vi "Calibration_user_input.vi"(4 "data mode":enum16{"Take new data point", "Refit Curve"}(ring), 6 "Mode":T4, 7 "Fixed n":bool, 8 "OK":T13, 9 "Sampling speeds":T5={"Samples /ch"=300, "Sampling Rate /ch (Hz)"=50.0} {"Sampling Rate /ch (Hz)" min=0 format="%.2f"; "Samples /ch" min=0 step=1}) -> (1 "Sampling speeds Output":T5={"Samples /ch"=300, "Sampling Rate /ch (Hz)"=50.0} {"Sampling Rate /ch (Hz)" min=0 format="%.2f"; "Samples /ch" min=0 step=1}, 2 "Fixed n out":bool, 3 "Temp":dbl=21.0 format="%.1fC", 5 "Abs Press":dbl=1013.0 format="%.1fmBar")   [LabVIEW 2022 SP3]
uses:
  Controls/ok_button.ctl
  Calib Channel Setup.ctl
  Controls/Cal_Inst_type.ctl
  Controls/Ref_Inst_type.ctl
  Calib_mode.ctl
  Controls/PWA_Data.ctl
  Controls/zeroableInst.ctl
  Controls/Meas input Cluster.ctl
  Controls/Inst_type.ctl
  Controls/portOrDev.ctl
  Controls/calType.ctl
  Controls/channelState.ctl
  File/Setup_Filetype.ctl
  ADAM Client/Sub VIs/ADAM Controls/Channel_names.ctl
  <vilib>/Utility/error.llb/Trim Whitespace One-Sided.vi
  Globals/Calib_global.vi
  Globals/Constants_global.vi
  Globals/Meas_global.vi
panel:
  in  "zeroable?":T1
  out "InstADAMChName":string
  in  "Select ADAM Instrument":bool
  in  "PWA Data":T2
  in  "Ref Instrument type":T3
  out "Info":string
  out "XW Angle Calib Present?":bool
  out "XW Velocity Calib Present?":bool
  in  "Edit temp and Press":bool
  out "2nd ref instrument":T6={"2nd Ref type"=enum."LDA", "2nd inst present"=TRUE}
  in  "Ref vel for angle calib":T7={"Ch"=4, "Off ch no"=0, "Calib filename"=path "", "Ref Instrument type"=enum."LDA", "DAQ System"="", "Port/Dev"=""} {"Off ch no" min=0 max=1; "Ch" min=0 max=50}
  out "Instrument type":T8=enum."Cross wire angle"
  in  "angle calib":T9(ring)
  in  "Reference instrument":T10={"Ch"=4, "Off ch no"=0, "Calib filename"=path "", "Ref Instrument type"=enum."Enter Value", "Device"="", "Port"=""} {"Off ch no" min=0 max=1; "Ch" min=0 max=50}
  in  "instrument to calibrate":T11(array[cluster])=[{"Ch No"=1, "Off ch no"=1, "Acquisition Plug in "="", "Port"=""}, {"Ch No"=2, "Off ch no"=1, "Acquisition Plug in "="", "Port"=""}] {"Off ch no" min=0 max=1; "Ch No" min=0 max=1000}
  in  "Instrument type":T8=enum."Pressure Transducer"
  out "Calib filename":path
  out "Ch & spans":T12[](array[typedef])=[{"Ch No"=1, "Var name"="Cross wire 1", "Device"="", "Port"=""}, {"Ch No"=2, "Var name"="Cross wire 2", "Device"="", "Port"=""}] {"Ch No" min=0 max=7}
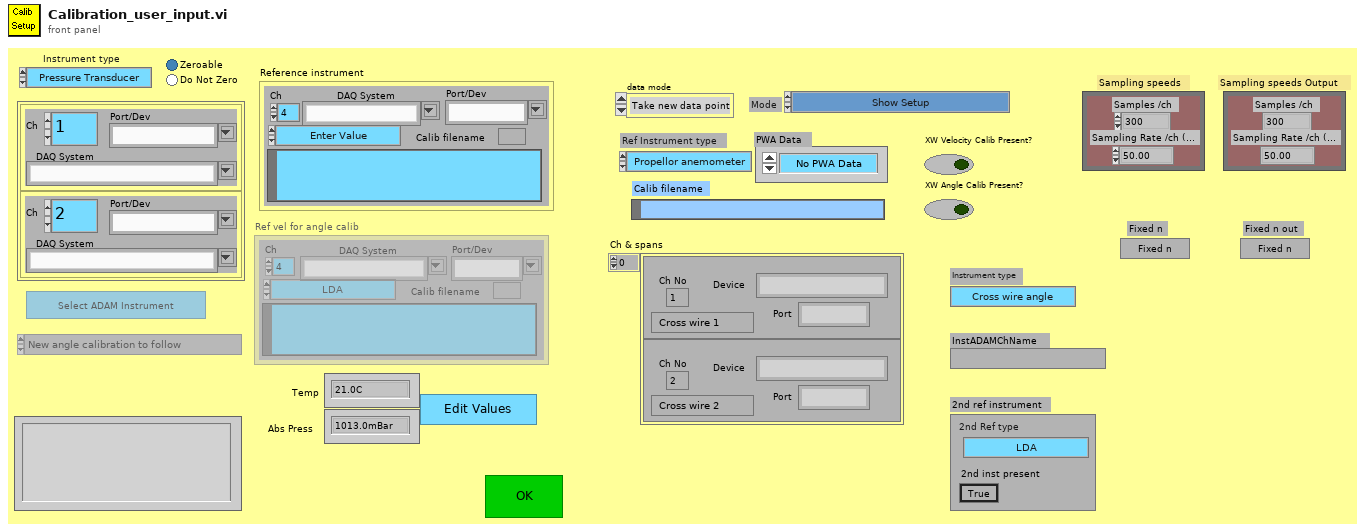
[diagram p1: front panel]
types:
  T1 = typedef "zeroableInst.ctl" = enum32{"Zeroable", "Do Not Zero"}
  T2 = typedef "PWA_Data.ctl" = enum16{"No PWA Data", "One Ch PWA"}
  T3 = typedef "Ref_Inst_type.ctl" = enum16{"Propellor anemometer", "Pressure Transducer", "Raw voltage", "Pitot-static tube", "Generic Linear", "Generic Polynomial", "Thermocouple", "LDA", "Enter Value", "ADAM Channel"}
  T4 = typedef "Calib_mode.ctl" = enum16{"Show Setup", "Take a New Calibration Point", "Refit Curve", "Setup Front Panel"}
  T5 = cluster{"Samples /ch":i32, "Sampling Rate /ch (Hz)":sgl}
  T6 = cluster{"2nd Ref type":T3, "2nd inst present":bool}
  T7 = cluster{"Ch":i16, "Off ch no":i8, "Calib filename":path, "Ref Instrument type":T3, "DAQ System":string, "Port/Dev":string}
  T8 = typedef "Cal_Inst_type.ctl" = enum16{"Propeller anemometer", "Pressure Transducer", "Hot wire", "Cross wire velocity", "Cross wire angle", "Generic Linear", "Generic Polynomial", "Poly Fit Special", "Fast FID", "Thermocouple", "Cold wire", "Pulsed Wire"}
  T9 = enum16{"New angle calibration to follow", "Use the most recent angle calibration"}
  T10 = cluster{"Ch":i16, "Off ch no":i8, "Calib filename":path, "Ref Instrument type":T3, "Device":string, "Port":string}
  T11 = cluster{"Ch No":i16, "Off ch no":i8, "Acquisition Plug in ":string, "Port":string}[]
  T12 = typedef "Calib Channel Setup.ctl" = cluster{"Ch No":i16, "Var name":string, "Device":string, "Port":string}
  T13 = typedef "ok_button.ctl" = bool
  T14 = typedef "Meas input Cluster.ctl" = cluster{"Type":T15, "Label":string, "DAQ":string, "Port":T16, "Ch":i32, "Cal":path, "calType":T17, "Fs":dbl, "syncDelay":dbl, "chState":T18}
  T15 = typedef "Inst_type.ctl" = enum16{"Raw voltage", "Raw with zero offsetting", "Propeller anemometer", "Pressure Transducer", "Pitot-static tube", "Hot wire", "Cross wire 1", "Cross wire 2", "Generic Linear", "Generic Polynomial", "Generic BackPoly", "Fast FID", "Thermocouple", "Cold wire", "Pulsed Wire", "LDA Vel", "LDA Tran time", "LDA Arr time", "Microphone"}
  T16 = typedef "portOrDev.ctl" = string
  T17 = typedef "calType.ctl" = enum32{"Latest", "Fixed"}
  T18 = typedef "channelState.ctl" = enum32{"No Selection", "Solo", "Mute"}
  T19 = typedef "Setup_Filetype.ctl" = enum16{"Measurement Setups", "Calibration Setups", "General", "Results File Plotter Setups", "Speed Calib Tweaks"}
  T20 = enum8{"Enabled", "Disabled", "Disabled and Grayed Out"}
  T21 = typedef "Channel_names.ctl" = enum16{"Active Only", "Active + Off", "All Channels", "Changeable Only", "Always Off", "Always On", "Always Off or On"}
  T22 = cluster{"Ch No":i16, "Off ch no":i8, "Device":string, "Port":string}[]
  T23 = cluster{"Ch No":i16, "Off ch no":i8, "Acquisition Plug in ":string, "Port":string}
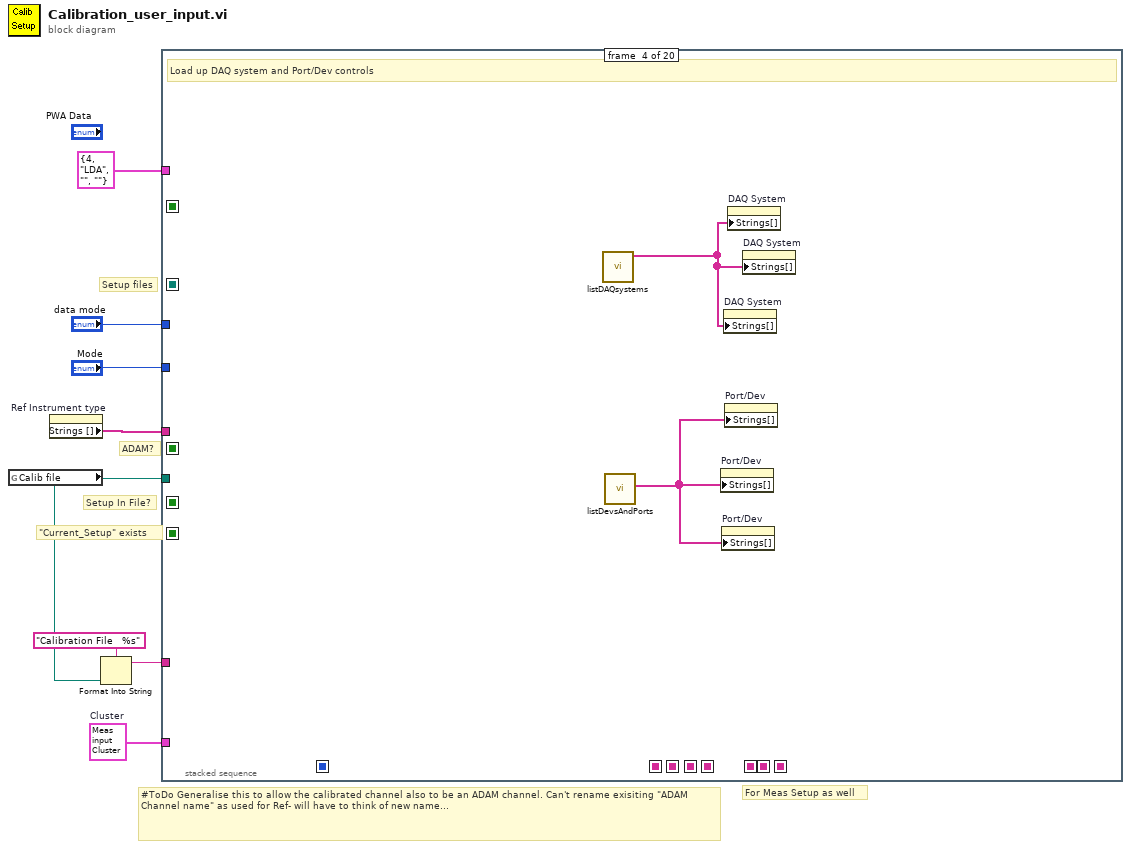
[diagram p0: block diagram]
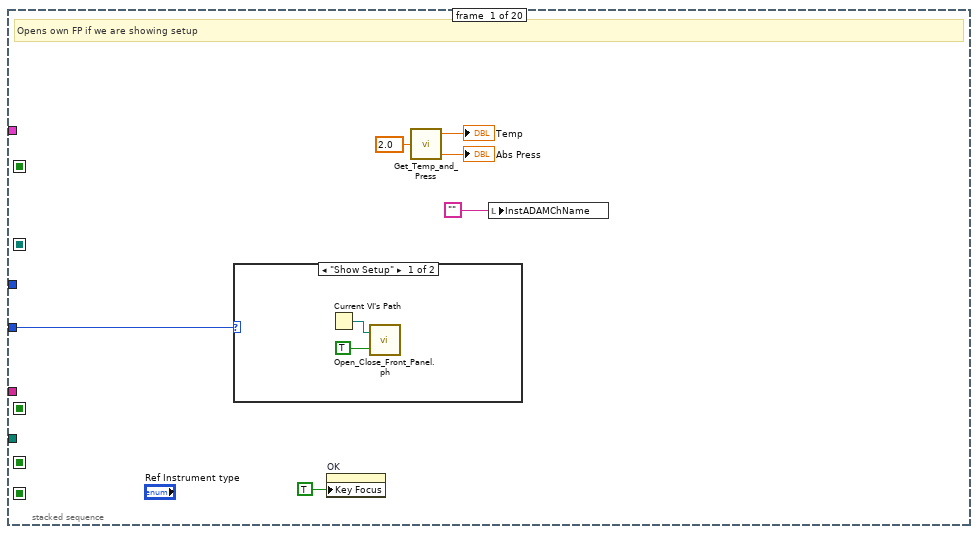
[diagram p2: hidden frame]
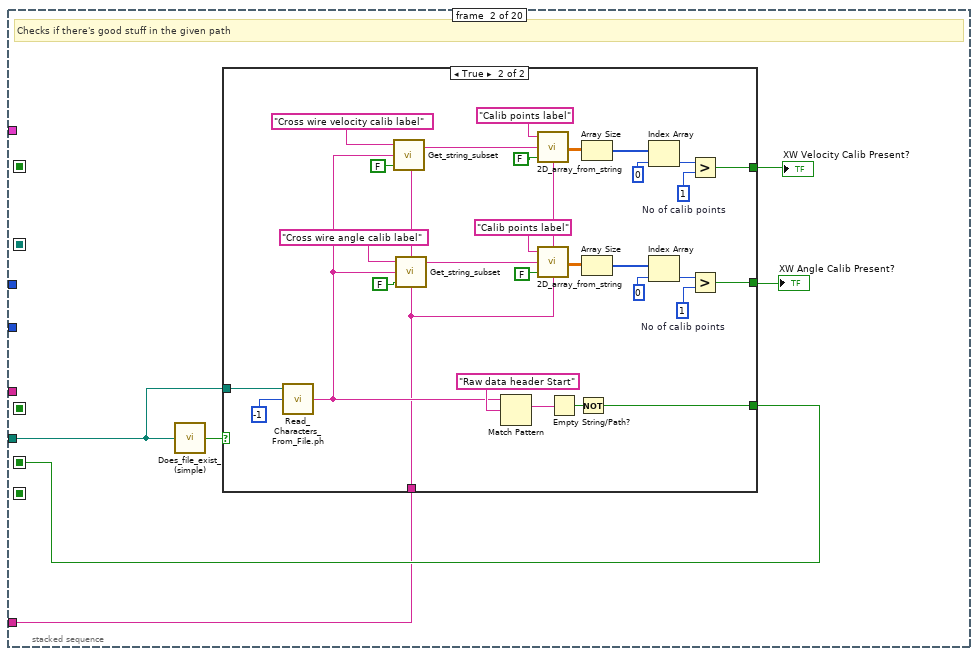
[diagram p4: hidden frame]
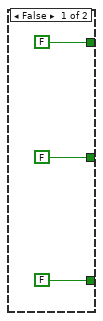
[diagram p5: hidden frame]
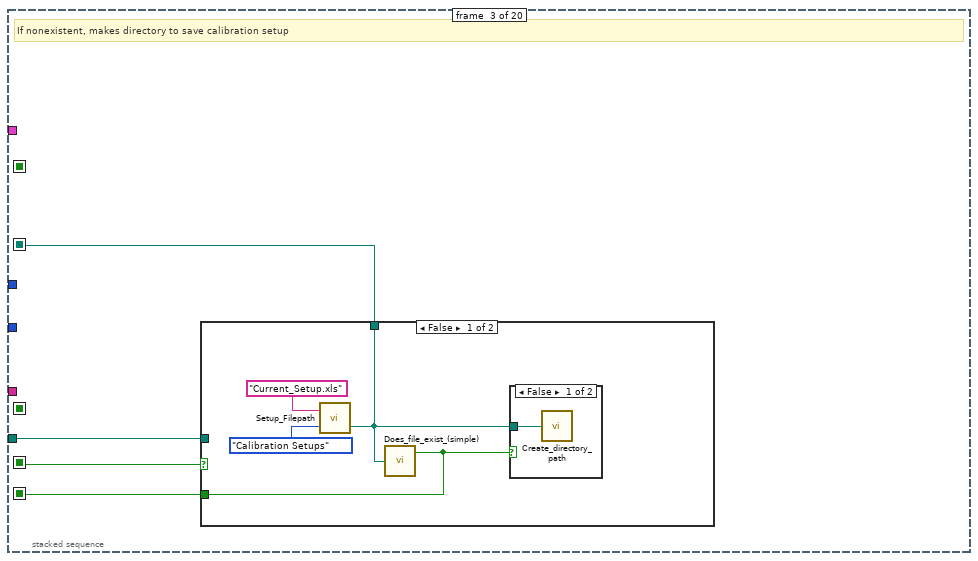
[diagram p6: hidden frame]
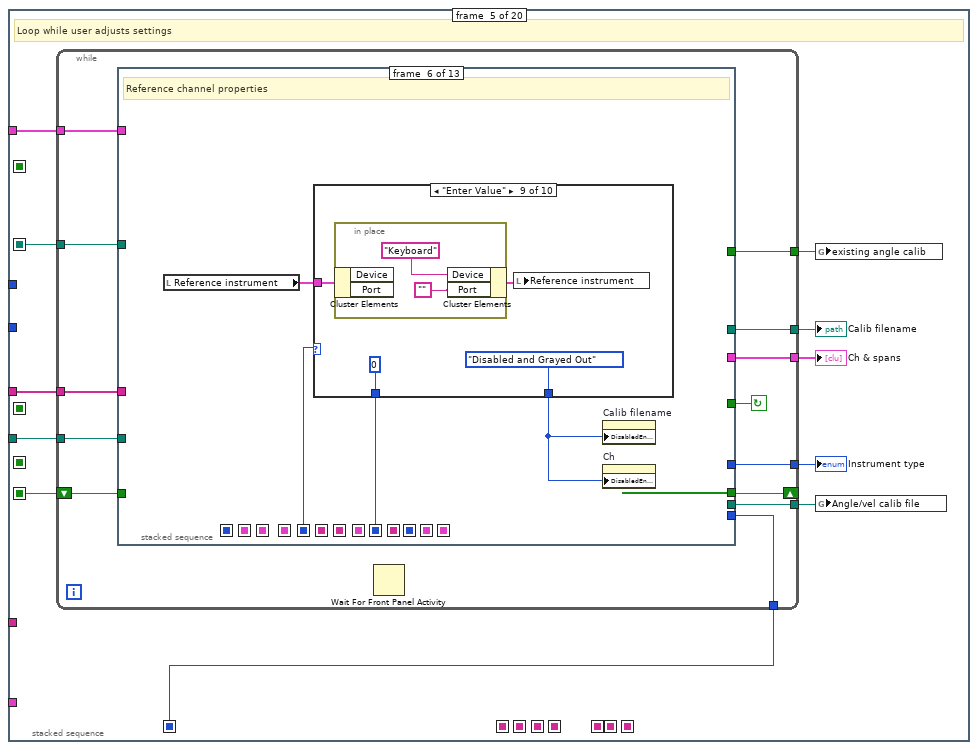
[diagram p9: hidden frame]
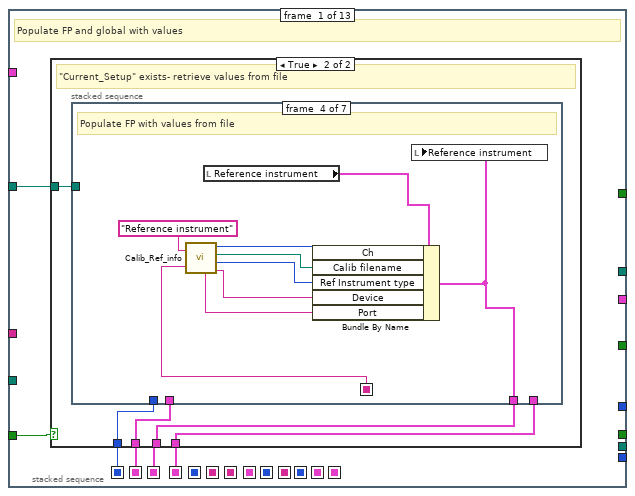
[diagram p10: hidden frame]
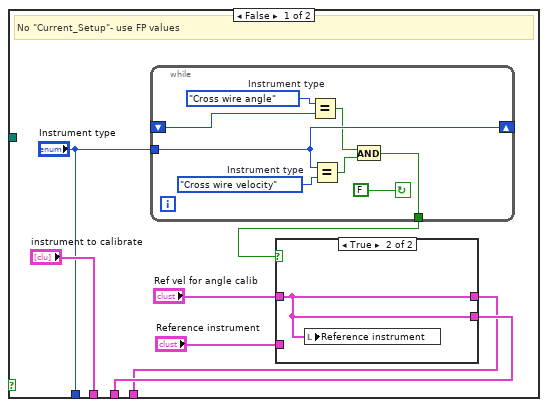
[diagram p11: hidden frame]
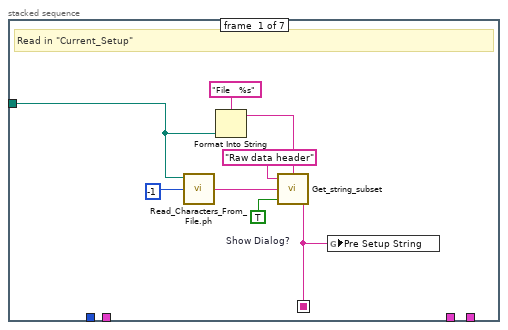
[diagram p13: hidden frame]
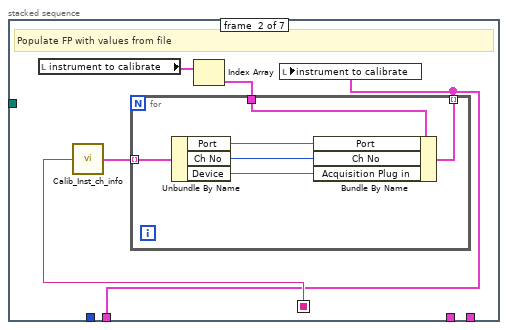
[diagram p14: hidden frame]
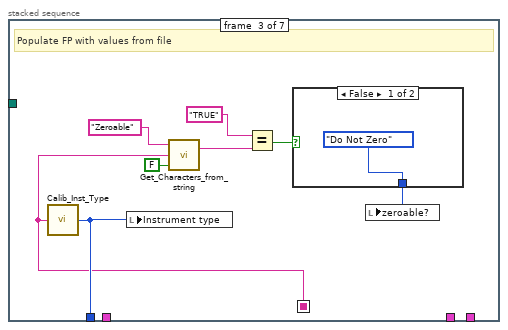
[diagram p15: hidden frame]
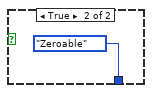
[diagram p16: hidden frame]
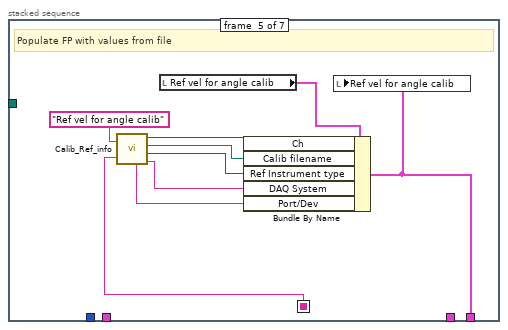
[diagram p17: hidden frame]
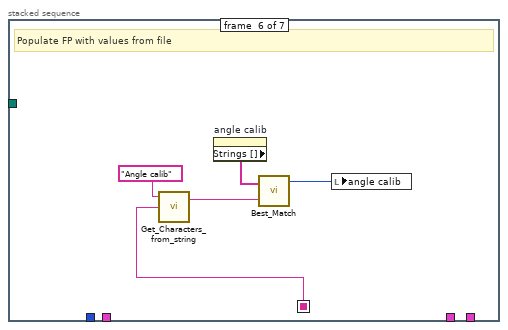
[diagram p18: hidden frame]
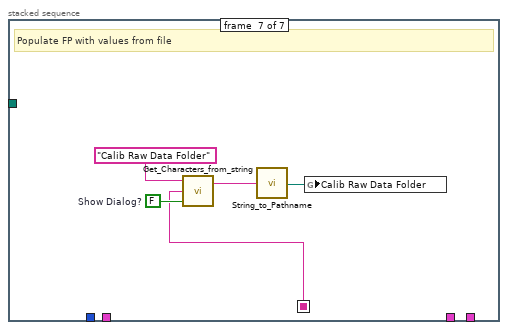
[diagram p19: hidden frame]
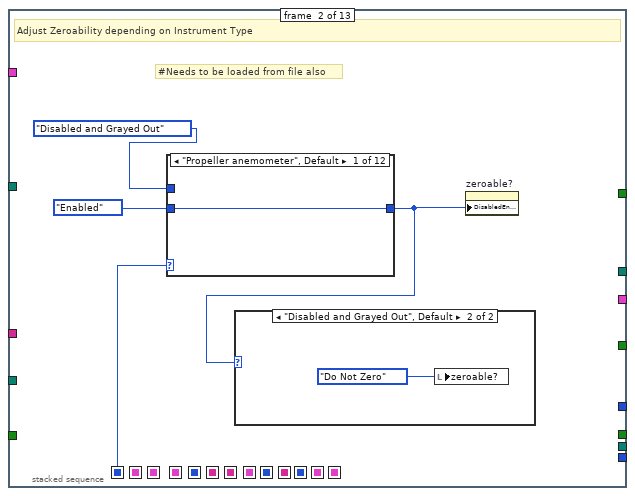
[diagram p20: hidden frame]
diagram:
  w1 = T14 {"Type"=enum."Raw voltage", "Label"="", "DAQ"="", "Port"="", "Ch"=0, "Cal"=path "", "calType"=enum."Latest", "Fs"=0.0, "syncDelay"=0.0, "chState"=enum."No Selection"}  # Cluster
  # "For Meas Setup as well"
  # "\"Current_Setup\" exists"
  # "#ToDo Generalise this to allow the calibrated channel also to be an ADAM channel. Can't rename exisiting \"ADAM Channel name\" as used for Ref- will have to think of new name..."
  # "Setup In File?"
  # "Setup files"
  # "ADAM?"
  n1 = global read "Calib_global.vi" "Calib file"() -> (w4:path)
  n2 = property on="Ref Instrument type" class="Enum (strict)"() -> ("Strings []"=w6:string[])  [unwired: 2 in, 2 out]
  n3 = Format Into String(format string="Calibration File   %s", w4) -> (resulting string=w3:string)  [unwired: 2 in, 1 out]
  n4 = stacked-sequence {
    seq-local: [_ _ w58 _ _ _ _ _ _ _ _ _ _ _ _ _ _ _ _ _] -> [_ _ _ _ w77 _ _ _ _ _ _ _ _ _ _ _ _ _ _ _]
    seq-local: [_ _ w59 _ _ _ _ _ _ _ _ _ _ _ _ _ _ _ _ _] -> [_ _ _ _ w75 _ _ _ _ _ _ _ _ _ _ _ _ _ _ _]
    seq-local: [_ _ _ _ w74 _ _ _ _ _ _ _ _ _ _ _ _ _ _ _] -> [_ _ _ _ _ _ _ _ w558 _ _ _ _ _ _ _ _ _ _ _]
    seq-local: [_ _ _ _ _ _ _ _ w559 _ _ _ _ _ _ _ _ _ _ _] -> [_ _ _ _ _ _ _ _ _ w576 _ _ _ _ _ _ _ _ _ _]
    seq-local: [_ _ _ _ _ _ _ _ _ w579 _ _ _ _ _ _ _ _ _ _] -> [_ _ _ _ _ _ _ _ _ _ _ _ _ _ _ _ w748 _ _ _]
    seq-local: [_ _ _ _ _ _ _ _ _ _ _ _ w649 _ _ _ _ _ _ _] -> [_ _ _ _ _ _ _ _ _ _ _ _ _ _ _ _ w747 _ w774 _]
    seq-local: [_ _ _ _ _ _ _ _ _ _ _ _ w647 _ _ _ _ _ _ _] -> [_ _ _ _ _ _ _ _ _ _ _ _ _ _ _ _ _ w755 _ _]
    seq-local: [_ w22 _ _ _ _ _ _ _ _ _ _ _ _ _ _ _ _ _ _] -> [_ _ w57 _ _ _ _ _ _ _ _ _ _ _ _ _ _ _ _ _]
    seq-local: [_ _ _ _ _ _ _ _ _ _ _ _ _ w671 _ _ _ _ _ _] -> [_ _ _ _ _ _ _ _ _ _ _ _ _ _ _ _ w740 _ _ _]
    seq-local: [_ _ _ _ _ _ _ _ _ _ _ _ _ _ _ w696 _ _ _ _] -> [_ _ _ _ _ _ _ _ _ _ _ _ _ _ _ _ w730 _ _ _]
    seq-local: [_ _ _ _ _ _ _ _ _ _ _ _ _ _ w678 _ _ _ _ _] -> [_ _ _ _ _ _ _ _ _ _ _ _ _ _ _ _ w729 _ w767 _]
    seq-local: [_ _ _ _ _ _ _ _ _ _ _ w612 _ _ _ _ _ _ _ _] -> [_ _ _ _ _ _ _ _ _ _ _ _ _ _ _ _ w728 _ _ _]
    seq-local: [_ _ _ _ _ _ _ _ _ _ w596 _ _ _ _ _ _ _ _ _] -> [_ _ _ _ _ _ _ _ _ _ _ _ _ _ _ _ w726 _ w763 _]
    tunnel: "Mode" -> [w10 _ _ _ _ w462 w483 _ _ w578 w604 w625 _ _ w679 _ _ w757 _ w794]
    tunnel: "data mode" -> [_ _ _ _ _ _ _ _ _ _ _ _ _ _ _ _ _ _ _ _]
    tunnel: w4 -> [_ w20 w56 _ w71 _ _ _ _ _ _ _ _ _ _ _ _ _ _ _]
    tunnel: w6 -> [_ _ _ _ w70 _ _ _ _ _ _ _ _ _ _ _ _ _ _ _]
    tunnel: w3 -> [_ w17 _ _ _ _ _ _ _ _ _ _ _ _ _ _ _ _ _ _]
    tunnel: T12 {"Ch No"=4, "Var name"="LDA", "Device"="", "Port"=""} ("Type") -> [_ _ _ _ w69 _ _ _ _ _ _ _ _ _ _ _ _ _ _ _]
    tunnel: w1 -> [_ _ _ _ _ _ w481 w522 _ _ _ _ _ _ _ _ _ _ _ _]
    frame #0 {
      # "Opens own FP if we are showing setup"
      n5 = case shown="\"Show Setup\"" w10 {
        frame "Show Setup" {
          n6 = Current VI's Path() -> (path=w16:path)
          n7 = call "Open_Close_Front_Panel.ph.vi"("openWindow (T)"=TRUE ("Front Panel Window:Open"), "VI path"=w16) -> ()  [unwired: 1 in, 1 out]
        }
        frame "Take a New Calibration Point", Default {
        }
      }
      n8 = property on="OK" class="Bool"("Key Focus"=TRUE) -> ()  [unwired: 2 in, 2 out]
      n9 = call "Get_Temp_and_Press.vi"("Averaging time (mins)"=2.0) -> ("Abs Press (mbar)"=→"Abs Press":dbl, "Temperature"=→"Temp":dbl)  [unwired: 3 out]
      n10 = local write "InstADAMChName"("") -> ()
    }
    frame #1 {
      # "Checks if there's good stuff in the given path"
      n11 = call "Does_file_exist_(simple).vi"("Pathname"=w20) -> ("exists?"=w21:bool)
      n12 = case shown="True" w21 {
        tunnel: [FALSE w51] -> w22
        tunnel: w20 -> [_ w50]
        tunnel: [FALSE w28] -> w19
        tunnel: [FALSE w27] -> w18
        tunnel: w17 -> [_ w26]
        frame False {
        }
        frame True {
          w39 = 1  # No of calib points
          w40 = 1  # No of calib points
          n13 = call "Read_Characters_From_File.ph.vi"("file path (dialog if empty)"=w50, "number of characters (all:-1)"=-1) -> ("character string"=w29:string)  [unwired: 7 out]
          n14 = call "Get_string_subset.vi"("String Name"=w26, "Show Dialog?"=FALSE, "String to split"=w29, "File Label"="Cross wire velocity calib label") -> ("Output string"=w37:string)  [unwired: 1 out]
          n15 = call "Get_string_subset.vi"("String Name"=w26, "Show Dialog?"=FALSE, "String to split"=w29, "File Label"="Cross wire angle calib label") -> ("Output string"=w42:string)  [unwired: 1 out]
          n16 = Match Pattern(string=w29, regular expression="Raw data header Start") -> (match substring=w53:string)  [unwired: 4 out]
          n17 = call "2D_array_from_string.vi"("String Name"=w26, "Show Dialog?"=FALSE, "Input string"=w37, "Array title"="Calib points label") -> ("2D data array"=w34:dbl[][])
          n18 = call "2D_array_from_string.vi"("String Name"=w26, "Show Dialog?"=FALSE, "Input string"=w42, "Array title"="Calib points label") -> ("2D data array"=w45:dbl[][])
          n19 = Empty String/Path?(string/path=w53) -> (empty?=w52:bool)
          n20 = Not(x=w52) -> (.not. x?=w51:bool)
          n21 = Array Size(array=w34) -> (size(s)=w35:i32[])
          n22 = Array Size(array=w45) -> (size(s)=w44:i32[])
          n23 = Index Array(array=w35, index=0 ("Index")) -> (element=w38:i32)
          n24 = Index Array(array=w44, index=0 ("Index")) -> (element=w41:i32)
          n25 = Greater?(x=w38, y=w39) -> (0:w27:bool)
          n26 = Greater?(x=w41, y=w40) -> (0:w28:bool)
        }
      }
      "XW Velocity Calib Present?" <- w18
      "XW Angle Calib Present?" <- w19
    }
    frame #2 {
      # "If nonexistent, makes directory to save calibration setup"
      n27 = case shown="False" w57 {
        tunnel: [w63 TRUE ("exists")] -> w59
        tunnel: [w60 w66] -> w58
        tunnel: w56 -> [_ w66]
        frame False {
          n28 = call "Setup_Filepath.vi"("Setup File Type"=Setup_Filetype."Calibration Setups", "Filename in"="Current_Setup.xls") -> ("Filename Out"=w60:path)  [unwired: 1 out]
          n29 = call "Does_file_exist_(simple).vi"("Pathname"=w60) -> ("exists?"=w63:bool)
          n30 = case shown="False" w63 {
            tunnel: w60 -> [w64 _]
            frame False {
              n31 = call "Create_directory_path.vi"("Path name"=w64) -> ()  [unwired: 2 in, 2 out]
            }
            frame True {
            }
          }
        }
        frame True {
        }
      }
    }
    frame #3 {
      # "Load up DAQ system and Port/Dev controls"
      n32 = call "listDAQsystems.vi"() -> ("DAQsystems"=w68:string[])  [unwired: 11 in]
      n33 = call "listDevsAndPorts.vi"() -> ("All Available Ports"=w67:string[])  [unwired: 11 in]
      n34 = property on="Port/Dev" class="CmbBox"("Strings[]"=w67) -> ()  [unwired: 2 in, 2 out]
      n35 = property on="Port/Dev" class="CmbBox"("Strings[]"=w67) -> ()  [unwired: 2 in, 2 out]
      n36 = property on="DAQ System" class="CmbBox"("Strings[]"=w68) -> ()  [unwired: 2 in, 2 out]
      n37 = property on="Port/Dev" class="CmbBox"("Strings[]"=w67) -> ()  [unwired: 2 in, 2 out]
      n38 = property on="DAQ System" class="CmbBox"("Strings[]"=w68) -> ()  [unwired: 2 in, 2 out]
      n39 = property on="DAQ System" class="CmbBox"("Strings[]"=w68) -> ()  [unwired: 2 in, 2 out]
    }
    frame #4 {
      # "Loop while user adjusts settings"
      n40 = while {
        tunnel: w70 -> [w83]
        shift-left: w75 -> [w86]
        shift-right: [w85] -> _
        tunnel: [w87] -> w76
        tunnel: w77 -> [w88]
        tunnel: [w89] -> w73
        tunnel: [w90] -> w79
        tunnel: [w91] -> w74
        tunnel: [w92] -> w78
        tunnel: [w82] -> w72
        tunnel: w71 -> [w81]
        tunnel: w69 -> [w80]
        stop <- w84 continue-if-true
        n41 = stacked-sequence {
          seq-local: [_ _ w201 _ _ _ _ _ _ _ _ _ _] -> [_ _ _ _ _ w307 _ _ _ _ _ _ _]
          seq-local: [_ _ w205 _ _ _ _ _ _ _ _ _ _] -> [_ _ _ _ _ _ _ _ w365 _ _ _ _]
          seq-local: [_ _ _ _ _ w306 _ _ _ _ _ _ _] -> [_ _ _ _ _ _ _ _ _ w382 _ _ _]
          seq-local: [_ _ w200 _ _ _ _ _ _ _ _ _ _] -> [_ _ _ _ _ _ _ _ _ w380 _ _ _]
          seq-local: [_ _ _ _ _ _ _ _ w364 _ _ _ _] -> [_ _ _ _ _ _ _ _ _ w381 _ _ _]
          seq-local: [_ _ _ _ _ _ _ w331 _ _ _ _ _] -> [_ _ _ _ _ _ _ _ _ w378 _ _ _]
          seq-local: [_ _ _ _ _ _ w324 _ _ _ _ _ _] -> [_ _ _ _ _ _ _ _ _ w377 _ _ _]
          seq-local: [w96 _ _ _ _ _ _ _ _ _ _ _ _] -> [_ w182 w203 w224 w238 _ _ w332 _ _ _ _ _]
          seq-local: [w95 _ _ _ _ _ _ _ _ _ _ _ _] -> [_ _ _ w223 _ _ _ _ _ _ w414 _ _]
          seq-local: [w94 _ _ _ _ _ _ _ _ _ _ _ _] -> [_ _ _ _ _ _ w326 w333 _ w376 _ _ _]
          seq-local: [w93 _ _ _ _ _ _ _ _ _ _ _ _] -> [_ _ w202 _ _ _ _ _ _ w375 _ _ _]
          seq-local: [_ _ _ _ _ _ _ _ _ w374 _ _ _] -> [_ _ _ _ _ _ _ _ _ _ _ _ w431]
          seq-local: [_ _ _ w219 _ _ _ _ _ _ _ _ _] -> [_ _ _ _ _ _ _ _ w363 _ _ _ _]
          tunnel: [_ _ _ _ _ _ _ _ _ w379 _ _ _] -> w92
          tunnel: [_ _ w201 _ _ _ _ _ _ _ _ _ _] -> w91
          tunnel: [_ _ _ _ _ _ _ _ _ w374 _ _ _] -> w90
          tunnel: [_ _ _ _ w242 _ _ _ _ _ _ _ _] -> w89
          tunnel: w88 -> [w98 _ _ _ _ _ _ _ _ _ _ _ _]
          tunnel: [_ _ w203 _ _ _ _ _ _ _ _ _ _] -> w87
          tunnel: w86 -> [w97 _ _ _ _ _ _ _ _ _ _ _ _]
          tunnel: [_ _ _ _ _ _ _ _ _ _ _ _ FALSE] -> w85
          tunnel: [_ _ _ _ _ _ _ _ _ _ _ _ w432] -> w84
          tunnel: w83 -> [_ _ w199 _ _ _ w323 _ _ _ _ _ _]
          tunnel: [_ _ _ _ w241 _ _ _ _ _ _ _ _] -> w82
          tunnel: w81 -> [_ _ _ _ w243 _ _ _ _ _ _ _ _]
          tunnel: w80 -> [_ _ _ _ _ _ _ _ w362 w373 _ _ _]
          frame #0 {
            # "Populate FP and global with values"
            n42 = case shown="True" w97 {
              tunnel: w98 -> [_ w121]
              tunnel: ["Instrument type" w119] -> w96
              tunnel: ["instrument to calibrate" w120] -> w95
              tunnel: [w100 w117] -> w94
              tunnel: [w102 w118] -> w93
              frame False {
                # "No \"Current_Setup\"- use FP values"
                n43 = while {
                  shift-right: [w114] -> _
                  shift-left: _ -> [w112]
                  tunnel: "Instrument type" -> [w114]
                  tunnel: [w109] -> w103
                  stop <- FALSE continue-if-true
                  w113 = Cal_Inst_type."Cross wire angle"  # Instrument type
                  w115 = Cal_Inst_type."Cross wire velocity"  # Instrument type
                  n44 = Equal?(x=w113, y=w112) -> (x = y?=w110:bool)
                  n45 = Equal?(x=w114, y=w115) -> (x = y?=w111:bool)
                  n46 = And(x=w110, y=w111) -> (x .and. y?=w109:bool)
                }
                n47 = case shown="True" w103 {
                  tunnel: [w107 w108] -> w102
                  tunnel: "Reference instrument" -> [w107 _]
                  tunnel: [w106 w108] -> w100
                  tunnel: "Ref vel for angle calib" -> [w106 w108]
                  frame False {
                  }
                  frame True {
                    n48 = local write "Reference instrument"(w108) -> ()
                  }
                }
              }
              frame True {
                # "\"Current_Setup\" exists- retrieve values from file"
                n49 = stacked-sequence {
                  seq-local: [w126 _ _ _ _ _ _] -> [_ w134 w143 w158 w164 w171 w176]
                  tunnel: w121 -> [w123 _ _ _ _ _ _]
                  tunnel: [_ w130 _ _ _ _ _] -> w120
                  tunnel: [_ _ w148 _ _ _ _] -> w119
                  tunnel: [_ _ _ w157 _ _ _] -> w118
                  tunnel: [_ _ _ _ w163 _ _] -> w117
                  frame #0 {
                    w125 = TRUE  # Show Dialog?
                    # "Read in \"Current_Setup\""
                    n50 = call "Read_Characters_From_File.ph.vi"("file path (dialog if empty)"=w123, "number of characters (all:-1)"=-1) -> ("character string"=w129:string)  [unwired: 7 out]
                    n51 = Format Into String(format string="File   %s", w123) -> (resulting string=w122:string)  [unwired: 2 in, 1 out]
                    n52 = call "Get_string_subset.vi"("String Name"=w122, "Show Dialog?"=w125, "String to split"=w129, "File Label"="Raw data header") -> ("Output string"=w126:string)  [unwired: 1 out]
                    n53 = global write "Calib_global.vi" "Pre Setup String"(w126) -> ()
                  }
                  frame #1 {
                    # "Populate FP with values from file"
                    n54 = local read "instrument to calibrate"() -> (w132:T11)
                    n55 = call "Calib_Inst_ch_info.vi"("Input string"=w134) -> ("instrument to calibrate"=w133:T22)
                    n56 = Index Array(array=w132) -> (element=w131:T23)  [unwired: 1 in]
                    n57 = for {
                      tunnel: w133 -> [w140] mode=indexing
                      tunnel: w131 -> [w139]
                      tunnel: [w137] -> w130 mode=indexing
                      n58 = Unbundle By Name(w140) -> ("Port"=w136:string, "Ch No"=w138:i16, "Device"=w135:string)
                      n59 = Bundle By Name(cluster=w139, "Port"=w136, "Ch No"=w138, "Acquisition Plug in"=w135) -> (w137:T23)
                    }
                    n60 = local write "instrument to calibrate"(w130) -> ()
                  }
                  frame #2 {
                    # "Populate FP with values from file"
                    n61 = call "Calib_Inst_Type.vi"("Input string"=w143) -> ("Instrument type"=w148:T8)
                    n62 = local write "Instrument type"(w148) -> ()
                    n63 = call "Get_Characters_from_string.vi"("Show Dialog?"=FALSE, "Input string"=w143, "Variable name"="Zeroable") -> ("Value"=w147:string)  [unwired: 1 out]
                    n64 = Equal?(x="TRUE", y=w147) -> (x = y?=w142:bool)
                    n65 = case shown="False" w142 {
                      tunnel: [zeroableInst."Do Not Zero" ("zeroable?") zeroableInst."Zeroable" ("zeroable?")] -> w141
                      frame False {
                      }
                      frame True {
                      }
                    }
                    n66 = local write "zeroable?"(w141) -> ()
                  }
                  frame #3 {
                    # "Populate FP with values from file"
                    n67 = call "Calib_Ref_info.vi"("Input string"=w158, "Reference Name"="Reference instrument") -> ("Device"=w151:string, "Ref Instrument type"=w154:T3, "Calib filename"=w155:path, "Ch No"=w156:i16, "Port"=w152:string)
                    n68 = local read "Reference instrument"() -> (w153:T10)
                    n69 = Bundle By Name(cluster=w153, "Ch"=w156, "Calib filename"=w155, "Ref Instrument type"=w154, "Device"=w151, "Port"=w152) -> (w157:T10)
                    n70 = local write "Reference instrument"(w157) -> ()
                  }
                  frame #4 {
                    # "Populate FP with values from file"
                    n71 = call "Calib_Ref_info.vi"("Input string"=w164, "Reference Name"="Ref vel for angle calib") -> ("Device"=w160:string, "Ref Instrument type"=w166:T3, "Calib filename"=w167:path, "Ch No"=w168:i16, "Port"=w161:string)
                    n72 = local read "Ref vel for angle calib"() -> (w162:T7)
                    n73 = Bundle By Name(cluster=w162, "Ch"=w168, "Calib filename"=w167, "Ref Instrument type"=w166, "DAQ System"=w160, "Port/Dev"=w161) -> (w163:T7)
                    n74 = local write "Ref vel for angle calib"(w163) -> ()
                  }
                  frame #5 {
                    # "Populate FP with values from file"
                    n75 = call "Get_Characters_from_string.vi"("Input string"=w171, "Variable name"="Angle calib") -> ("Value"=w170:string)  [unwired: 1 in, 1 out]
                    n76 = property on="angle calib" class="Enum (strict)"() -> ("Strings []"=w173:string[])  [unwired: 2 in, 2 out]
                    n77 = call "Best_Match.vi"("Input String"=w170, "String Options"=w173) -> ("index of element"=w169:i32)  [unwired: 1 out]
                    n78 = local write "angle calib"(w169) -> ()
                  }
                  frame #6 {
                    w177 = FALSE  # Show Dialog?
                    # "Populate FP with values from file"
                    n79 = call "Get_Characters_from_string.vi"("Show Dialog?"=w177, "Input string"=w176, "Variable name"="Calib Raw Data Folder") -> ("Value"=w175:string)  [unwired: 1 out]
                    n80 = call "String_to_Pathname.vi"("Input String"=w175) -> ("path"=w174:path)
                    n81 = global write "Calib_global.vi" "Calib Raw Data Folder"(w174) -> ()
                  }
                }
              }
            }
          }
          frame #1 {
            # "#Needs to be loaded from file also"
            # "Adjust Zeroability depending on Instrument Type"
            n82 = case shown="\"Propeller anemometer\", Default" w182 {
              tunnel: [w184 w185 w186 w187 w188 w189 w190 w191 w192 w193 w194 w195] -> w179
              tunnel: T20."Enabled" ("Disabled") -> [w184 w185 _ _ _ w189 w190 w191 _ _ _ _]
              tunnel: T20."Disabled and Grayed Out" ("Disabled") -> [_ _ w186 w187 w188 _ _ _ w192 w193 w194 w195]
              frame "Propeller anemometer", Default {
              }
              frame "Pressure Transducer" {
              }
              frame "Hot wire" {
              }
              frame "Cross wire velocity" {
              }
              frame "Cross wire angle" {
              }
              frame "Generic Linear" {
              }
              frame "Generic Polynomial" {
              }
              frame "Poly Fit Special" {
              }
              frame "Fast FID" {
              }
              frame "Thermocouple" {
              }
              frame "Cold wire" {
              }
              frame "Pulsed Wire" {
              }
            }
            n83 = case shown="\"Disabled and Grayed Out\", Default" w179 {
              frame "Enabled" {
              }
              frame "Disabled and Grayed Out", Default {
                n84 = local write "zeroable?"(zeroableInst."Do Not Zero" ("zeroable?")) -> ()
              }
            }
            n85 = property on="zeroable?" class="RadioBtnsControl (strict)"("DisabledEnum"=w179) -> ()  [unwired: 2 in, 2 out]
          }
          frame #2 {
            n86 = Unbundle By Name(w202) -> ("Ref Instrument type"=w204:T3)
            n87 = Build Array("Raw voltage", "Raw voltage") -> (w196:string[])
            n88 = case shown="\"Cross wire angle\"" w203 {
              tunnel: [w206 w208 w217] -> w205
              tunnel: w204 -> [w207 w209 w216]
              tunnel: [w207 w210 w216] -> w201
              tunnel: w202 -> [_ w211 _]
              tunnel: w196 -> [w206 w208 _]
              frame "Cross wire velocity" {
              }
              frame "Cross wire angle" {
                n89 = case shown="\"LDA\", Default" w209 {
                  selector: w209 -> [w213 w214 _]
                  tunnel: [w213 w214 Ref_Inst_type."Enter Value" ("Ref Instrument type")] -> w210
                  frame "Enter Value" {
                  }
                  frame "ADAM Channel" {
                  }
                  frame "LDA", Default {
                  }
                }
                n90 = Bundle By Name(cluster=w211, "Ref Instrument type"=w210) -> (w212:T10)
                n91 = local write "Reference instrument"(w212) -> ()
              }
              frame "Generic Linear", Default {
                n92 = Build Array("Raw voltage") -> (w217:string[])
              }
            }
            n93 = Index Array(array=w199, index=w201) -> (element=w200:string)
          }
          frame #3 {
            # "How many channels does Instrument comprise?"
            n94 = Array Size(array=w223) -> (size(s)=w222:i32)
            n95 = case shown="\"Cross wire angle\"" w224 {
              tunnel: [2 2 1 0] -> w221
              frame "Cross wire velocity" {
              }
              frame "Cross wire angle" {
              }
              frame "Generic Linear", Default {
              }
              frame "Pulsed Wire" {
              }
            }
            n96 = Equal?(x=w221, y=w222) -> (x = y?=w220:bool)
            n97 = case shown="False" w220 {
              tunnel: w221 -> [w230 _]
              tunnel: w223 -> [w226 w232]
              tunnel: [w225 w232] -> w219
              frame False {
                # "Multi-channel instrument"
                n98 = Index Array(array=w226, index=0) -> (element=w227:T23)
                n99 = Build Array (concatenate)(w226, w227) -> (w229:T11)
                n100 = for {
                  N: w230 -> [_]
                  tunnel: w229 -> [w231] mode=indexing
                  tunnel: [w231] -> w225 mode=indexing
                }
                n101 = local write "instrument to calibrate"(w225) -> ()
              }
              frame True {
                # "Regular single-channel instrument"
              }
            }
          }
          frame #4 {
            n102 = case shown="\"Cross wire velocity\"" w238 {
              selector: w238 -> [_ w250 w271]
              tunnel: w243 -> [_ w253 w275]
              tunnel: [path "" w254 w276] -> w242
              tunnel: [FALSE w252 w274] -> w241
              tunnel: [w244 T20."Enabled" ("Disabled") T20."Disabled and Grayed Out" ("Disabled")] -> w237
              tunnel: [w244 T20."Disabled and Grayed Out" ("Disabled") w273] -> w240
              tunnel: ["" w251 w272] -> w239
              frame "Propeller anemometer", Default {
                w244 = T20."Disabled and Grayed Out" ("Disabled")
              }
              frame "Cross wire angle" {
                n103 = local read "XW Velocity Calib Present?"() -> (w255:bool)
                n104 = case shown="False" w255 {
                  tunnel: [w259 w269] -> w254
                  tunnel: w253 -> [_ w269]
                  tunnel: [TRUE TRUE] -> w252
                  tunnel: [w257 "Will use the velocity Calibration info already in the Calibration file. " ("resulting string")] -> w251
                  tunnel: w250 -> [w256 _]
                  frame False {
                    n105 = local read "instrument to calibrate"() -> (w264:T11)
                    n106 = Index Array(array=w264, index=0) -> (element=w262:T23)
                    n107 = Unbundle By Name(w262) -> ("Ch No"=w260:i16)
                    n108 = call "XW_file_info.vi"("Instrument type"=w256, "Ch No"=w260) -> ("Filename"=w259:path, "resulting string"=w257:string, "File Exists?"=w258:bool)
                    n109 = case shown="False" w258 {
                      frame False {
                        w265 = Cal_Inst_type."Cross wire velocity"  # Instrument type
                        n110 = local write "Instrument type"(w265) -> ()
                        n111 = One Button Dialog(message="You need to do a velocity calibration before you can do the angle calibration") -> ()  [unwired: 2 out]
                      }
                      frame True {
                      }
                    }
                  }
                  frame True {
                  }
                }
              }
              frame "Cross wire velocity" {
                n112 = local read "XW Angle Calib Present?"() -> (w277:bool)
                n113 = case shown="False" w277 {
                  tunnel: [w286 w303] -> w276
                  tunnel: w275 -> [_ w303]
                  tunnel: [w285 TRUE] -> w274
                  tunnel: [w284 T20."Enabled" ("Disabled")] -> w273
                  tunnel: [w280 "Will use the angle Calibration info already in the Calibration file. " ("resulting string")] -> w272
                  tunnel: w271 -> [w278 _]
                  frame False {
                    n114 = local read "instrument to calibrate"() -> (w290:T11)
                    n115 = Index Array(array=w290, index=0) -> (element=w288:T23)
                    n116 = Unbundle By Name(w288) -> ("Ch No"=w283:i16)
                    n117 = call "XW_file_info.vi"("Instrument type"=w278, "Ch No"=w283) -> ("Filename"=w282:path, "resulting string"=w279:string, "File Exists?"=w281:bool)
                    n118 = case shown="\"New angle calibration to follow\"" "angle calib" {
                      tunnel: [path "" w296] -> w286
                      tunnel: w282 -> [_ w296]
                      tunnel: [FALSE TRUE] -> w285
                      tunnel: ["This XW velocity Calibration MUST be followed by an angle calibration, before XW measurements can be made." w294] -> w280
                      tunnel: w279 -> [_ w294]
                      frame "New angle calibration to follow" {
                      }
                      frame "Use the most recent angle calibration" {
                      }
                    }
                    n119 = case shown="False" w281 {
                      tunnel: [T20."Disabled and Grayed Out" ("Disabled") T20."Enabled" ("Disabled")] -> w284
                      frame False {
                        n120 = local write "angle calib"(T9."New angle calibration to follow" ("angle calib")) -> ()
                      }
                      frame True {
                      }
                    }
                  }
                  frame True {
                  }
                }
              }
            }
            "Info" <- w239
            n121 = property on="Ref vel for angle calib" class="Clust (strict)"("Disabled"=w237) -> ()  [unwired: 2 in, 2 out]
            n122 = property on="angle calib" class="Enum (strict)"("Disabled"=w240) -> ()  [unwired: 2 in, 2 out]
          }
          frame #5 {
            # "Reference channel properties"
            n123 = local read "Reference instrument"() -> (w305:T10)
            n124 = case shown="\"Enter Value\"" w307 {
              tunnel: [1 1 1 1 1 1 0 0 0 0] -> w306
              tunnel: w305 -> [_ _ _ _ _ _ _ _ w318 _]
              tunnel: [_ _ _ _ _ _ _ _ T20."Disabled and Grayed Out" ("Disabled") _] -> w304
              frame "Propellor anemometer" {
              }
              frame "Pressure Transducer" {
              }
              frame "Raw voltage" {
              }
              frame "Pitot-static tube" {
              }
              frame "Generic Linear" {
              }
              frame "Generic Polynomial" {
              }
              frame "Thermocouple" {
              }
              frame "LDA" {
              }
              frame "Enter Value" {
                n125 = in-place {
                  n126 = in-place-cluster #1(w318) -> ()  [unwired: 2 out]
                  n127 = in-place-cluster #1("Device"="Keyboard", "Port"="") -> (w317:T10)
                }
                n128 = local write "Reference instrument"(w317) -> ()
              }
              frame "ADAM Channel" {
              }
            }
            n129 = property on="Calib filename" class="Path"("DisabledEnum"=w304) -> ()  [unwired: 2 in, 2 out]
            n130 = property on="Ch" class="DigNum (strict)"("DisabledEnum"=w304) -> ()  [unwired: 2 in, 2 out]
          }
          frame #6 {
            n131 = Unbundle By Name(w326) -> ("Ref Instrument type"=w325:T3)
            n132 = Index Array(array=w323, index=w325) -> (element=w324:string)
          }
          frame #7 {
            # "Add 2nd ref if required by ref type and X wire"
            n133 = Unbundle By Name(w333) -> ("Ref Instrument type"=w334:T3)
            n134 = case shown="\"Raw voltage\"" w334 {
              tunnel: [w341 w343 w346 w348 w350 w352 w354 w356 w358 w360] -> w335
              tunnel: [w341 w343 w345 w348 w350 w352 w354 w356 w358 w360] -> w329
              tunnel: [w341 w343 w346 w348 w350 w352 w354 w356 w358 w360] -> w338
              tunnel: [w341 w343 w346 w348 w350 w352 w354 w356 w358 w360] -> w337
              tunnel: [w341 w343 w346 w348 w350 w352 w354 w356 w358 w360] -> w336
              tunnel: [enum16{"No 2nd ref inst", "Add 2nd ref inst"}."Add 2nd ref inst" enum16{"No 2nd ref inst", "Add 2nd ref inst"}."Add 2nd ref inst" enum16{"No 2nd ref inst", "Add 2nd ref inst"}."Add 2nd ref inst" enum16{"No 2nd ref inst", "Add 2nd ref inst"}."Add 2nd ref inst" enum16{"No 2nd ref inst", "Add 2nd ref inst"}."Add 2nd ref inst" enum16{"No 2nd ref inst", "Add 2nd ref inst"}."Add 2nd ref inst" enum16{"No 2nd ref inst", "Add 2nd ref inst"}."Add 2nd ref inst" enum16{"No 2nd ref inst", "Add 2nd ref inst"}."No 2nd ref inst" enum16{"No 2nd ref inst", "Add 2nd ref inst"}."No 2nd ref inst" enum16{"No 2nd ref inst", "Add 2nd ref inst"}."No 2nd ref inst"] -> w330
              tunnel: T20."Enabled" ("Disabled") -> [w341 w343 w346 w348 w350 w352 w354 _ _ _]
              tunnel: T20."Disabled and Grayed Out" ("Disabled") -> [_ _ w345 _ _ _ _ w356 w358 w360]
              frame "Propellor anemometer" {
              }
              frame "Pressure Transducer" {
              }
              frame "Raw voltage" {
              }
              frame "Pitot-static tube" {
              }
              frame "Generic Linear" {
              }
              frame "Generic Polynomial" {
              }
              frame "Thermocouple" {
              }
              frame "LDA" {
              }
              frame "Enter Value" {
              }
              frame "ADAM Channel" {
              }
            }
            n135 = case shown="\"Cross wire angle\"" w332 {
              tunnel: [w339 enum16{"No 2nd ref inst", "Add 2nd ref inst"}."No 2nd ref inst"] -> w331
              tunnel: w330 -> [w339 _]
              frame "Cross wire angle" {
              }
              frame "Generic Linear", Default {
              }
            }
            n136 = property on="Off ch no" class="DigNum (strict)"("Disabled"=w338) -> ()  [unwired: 2 in, 2 out]
            n137 = property on="Calib filename" class="Path"("DisabledEnum"=w329) -> ()  [unwired: 2 in, 2 out]
            n138 = property on="Ch" class="DigNum (strict)"("Disabled"=w337) -> ()  [unwired: 2 in, 2 out]
            n139 = property on="Calib filename" class="Path"("Disabled"=w336) -> ()  [unwired: 2 in, 2 out]
            n140 = property on="Ref Instrument type" class="Enum (strict)"("Disabled"=w335) -> ()  [unwired: 2 in, 2 out]
          }
          frame #8 {
            # "Build Channel clusters"
            n141 = for {
              tunnel: w365 -> [w372] mode=indexing
              tunnel: [w371] -> w364 mode=indexing
              tunnel: w363 -> [w369] mode=indexing
              tunnel: w362 -> [w368]
              n142 = Unbundle By Name(w369) -> ("Acquisition Plug in"=w366:string, "Port"=w367:string, "Ch No"=w370:i16)
              n143 = Bundle By Name(cluster=w368, "Device"=w366, "Port"=w367, "Ch No"=w370, "Var name"=w372) -> (w371:T12)
            }
          }
          frame #9 {
            # "Append additional reference channels"
            n144 = case shown="1.." w382 {
              tunnel: [w386 w410] -> w374
              tunnel: w381 -> [w389 w404]
              tunnel: w375 -> [_ w407]
              tunnel: w380 -> [_ w406]
              tunnel: [w388 w409] -> w379
              tunnel: w373 -> [w387 w408]
              tunnel: w376 -> [w383 _]
              tunnel: w378 -> [w385 _]
              tunnel: w377 -> [w384 _]
              frame ..0 {
                n145 = case shown="\"No 2nd ref inst\"" w385 {
                  tunnel: [w391 w401] -> w386
                  tunnel: w384 -> [_ w400]
                  tunnel: w383 -> [_ w399]
                  tunnel: w387 -> [_ w398]
                  tunnel: [path "" w397] -> w388
                  tunnel: w389 -> [w391 w394]
                  frame "No 2nd ref inst" {
                  }
                  frame "Add 2nd ref inst" {
                    n146 = Unbundle By Name(w399) -> ("DAQ System"=w392:string, "Port/Dev"=w393:string, "Ch"=w396:i16, "Calib filename"=w397:path)
                    n147 = Bundle By Name(cluster=w398, "Device"=w392, "Port"=w393, "Ch No"=w396, "Var name"=w400) -> (w395:T12)
                    n148 = Build Array (concatenate)(w395, w394) -> (w401:T12[])
                  }
                }
              }
              frame 1.. {
                n149 = Unbundle By Name(w407) -> ("Device"=w402:string, "Port"=w403:string, "Ch"=w411:i16, "Calib filename"=w409:path)
                n150 = Bundle By Name(cluster=w408, "Device"=w402, "Port"=w403, "Ch No"=w411, "Var name"=w406) -> (w405:T12)
                n151 = Build Array (concatenate)(w405, w404) -> (w410:T12[])
              }
            }
          }
          frame #10 {
            n152 = Index Array(array=w414) -> (element=w413:T23)  [unwired: 1 in]
            n153 = Unbundle By Name(w413) -> ("Acquisition Plug in"=w412:string)
            n154 = Match Pattern(string=w412, regular expression="ADAM") -> (match substring=w416:string)  [unwired: 1 in, 3 out]
            n155 = case shown="\"ADAM\"" w416 {
              tunnel: "Select ADAM Instrument" -> [_ w419]
              frame "False", Default {
                n156 = property on="Select ADAM Instrument" class="Bool (strict)"("DisabledEnum"=T20."Disabled and Grayed Out" ("Disabled")) -> ()  [unwired: 2 in, 2 out]
              }
              frame "ADAM" {
                n157 = case shown="True" w419 {
                  frame False {
                  }
                  frame True {
                    n158 = local write "Select ADAM Instrument"(FALSE) -> ()
                    n159 = call "Get_ADAM_Ch_names_client.vi"("Channel names set"=Channel_names."Active Only") -> ("Ch names"=w423:string[])
                    n160 = call "Select_Single_ADAM_Ch.vi"("Available Ch names"=w423, "Message"="Please Choose ADAM Channel to calibrate") -> ("Ch Name"=→"InstADAMChName":string)  [unwired: 1 in, 3 out]
                  }
                }
                n161 = property on="Select ADAM Instrument" class="Bool (strict)"("DisabledEnum"=T20."Enabled" ("Disabled")) -> ()  [unwired: 2 in, 2 out]
              }
            }
          }
          frame #11 {
            # "Throw T/P panel if requested"
            n162 = case shown="True" "Edit temp and Press" {
              frame False {
              }
              frame True {
                n163 = stacked-sequence {
                  frame #0 {
                    w427 = TRUE  # Wait until done
                    n164 = call "Run_Enter_Temp.vi"("Wait until done"=w427) -> ()  [unwired: 1 out]
                  }
                  frame #1 {
                    n165 = call "Get_Temp_and_Press.vi"("Averaging time (mins)"=0.5) -> ("Abs Press (mbar)"=w429:dbl, "Temperature"=w428:dbl)  [unwired: 3 out]
                    n166 = local write "Abs Press"(w429) -> ()
                    n167 = local write "Temp"(w428) -> ()
                  }
                }
              }
            }
          }
          frame #12 {
            # "Check for \"OK\". Continue looping if any channel range/ name errors"
            n168 = case shown="True" "OK" {
              tunnel: w431 -> [_ w439]
              tunnel: [TRUE w437] -> w432
              frame False {
              }
              frame True {
                n169 = for {
                  shift-right: [w450] -> _
                  shift-left: string[] [] -> [w449]
                  tunnel: w439 -> [w447] mode=indexing
                  tunnel: [w446] -> w438 mode=indexing
                  n170 = Unbundle By Name(w447) -> ("Device"=w443:string, "Port"=w442:string, "Ch No"=w441:i16)
                  n171 = Format Into String(format string=" %s Ch %d", initial string=w443, w442, w441) -> (resulting string=w445:string)  [unwired: 1 in, 1 out]
                  n172 = call <vilib>:"Trim Whitespace.vi"("string"=w445) -> ("trimmed string"=w440:string)  [unwired: 1 in]
                  n173 = Search 1D Array(1D array=w449, element=w440) -> (index of element=w448:i32)  [unwired: 1 in]
                  n174 = Build Array (concatenate)(w449, w440) -> (w450:string[])
                  n175 = case shown="0, Default" w448 {
                    tunnel: w440 -> [w455 _]
                    tunnel: [w451 FALSE ("true")] -> w446
                    frame 0, Default {
                      n176 = Format Into String(format string="The Channel %s appears more than once", w455) -> (resulting string=w453:string)  [unwired: 2 in, 1 out]
                      n177 = One Button Dialog(message=w453, button name ("OK")="Ok") -> (true=w451:bool)
                    }
                    frame -1 {
                    }
                  }
                }
                n178 = Or Array Elements(Boolean array=w438) -> (logical OR=w437:bool)
              }
            }
          }
        }
        n179 = Wait For Front Panel Activity() -> ()  [unwired: 3 in, 1 out]
      }
      "Instrument type" <- w76
      "Ch & spans" <- w79
      "Calib filename" <- w78
      n180 = global write "Calib_global.vi" "existing angle calib"(w72) -> ()
      n181 = global write "Calib_global.vi" "Angle/vel calib file"(w73) -> ()
    }
    frame #5 {
      n182 = global read "Calib_global.vi" "Pre Setup String"() -> (w457:string)
      n183 = case shown="\"Setup Front Panel\"" w462 {
        tunnel: [w464 w477] -> w461
        tunnel: "Sampling speeds" -> [w464 w478]
        tunnel: [w463 w473] -> w459
        tunnel: "Fixed n" -> [w463 _]
        tunnel: w457 -> [_ w465]
        frame "Show Setup", Default {
        }
        frame "Setup Front Panel" {
          n184 = call "Get_value_from_string.vi"("Input string"=w465, "Variable name"="Requested sampling rate") -> ("Status"=w471:enum16{"Char in string", "Char not in string"}, "Value"=w470:dbl)  [unwired: 1 in]
          n185 = case shown="\"Char in string\"" w471 {
            tunnel: [w479 sgl 100.0 ("Sampling Rate /ch (Hz)")] -> w468
            tunnel: w470 -> [w479 _]
            frame "Char in string" {
            }
            frame "Char not in string" {
            }
          }
          n186 = call "Get_value_from_string.vi"("Input string"=w465, "Variable name"="Time per Block (s)") -> ("Value"=w467:dbl)  [unwired: 1 in, 1 out]
          n187 = call "Get_Characters_from_string.vi"("Input string"=w465, "Variable name"="Fixed Coefficient n") -> ("Value"=w475:string)  [unwired: 1 in, 1 out]
          n188 = Multiply(x=w467, y=w468) -> (x*y=w466:dbl)
          n189 = Bundle By Name(cluster=w478, "Samples /ch"=w466, "Sampling Rate /ch (Hz)"=w468) -> (w477:T5)
          n190 = Equal?(x="TRUE", y=w475) -> (x = y?=w473:bool)
        }
      }
      "Sampling speeds Output" <- w461
      "Fixed n out" <- w459
    }
    frame #6 {
      # "Get reference instrument calibration"
      n191 = local read "Reference instrument"() -> (w485:T10)
      n192 = property on="Calib filename" class="Path"() -> ("DisabledEnum"=w482:T20)  [unwired: 2 in, 2 out]
      n193 = Equal To 0?(x=w482) -> (x = 0?=w486:bool)
      n194 = case shown="True" w486 {
        tunnel: w485 -> [w489 w504]
        tunnel: [w488 w503] -> w484
        tunnel: w483 -> [_ w500]
        tunnel: w481 -> [_ w490]
        frame False {
          n195 = Bundle By Name(cluster=w489, "Calib filename"=path "") -> (w488:T10)
        }
        frame True {
          n196 = global read "Meas_global.vi" "Acquisition_Plug_Ins to Run"() -> (w495:string[])
          n197 = Unbundle By Name(w504) -> ("Ref Instrument type"=w502:T3, "Calib filename"=w499:path, "Ch"=w491:i16)
          n198 = global read "Calib_global.vi" "Pre Setup String"() -> (w497:string)
          n199 = case shown="\"Generic Linear\"" w502 {
            tunnel: [Inst_type."Propeller anemometer" ("Inst type") Inst_type."Pressure Transducer" ("Inst type") Inst_type."Pressure Transducer" ("Inst type") Inst_type."Pitot-static tube" ("Inst type") Inst_type."Generic Linear" ("Inst type") Inst_type."Generic Polynomial" ("Inst type") Inst_type."Thermocouple" ("Inst type") Inst_type."Raw voltage" ("Inst type") Inst_type."Raw voltage" ("Inst type") Inst_type."Raw voltage" ("Inst type")] -> w501
            frame "Propellor anemometer" {
            }
            frame "Pressure Transducer" {
            }
            frame "Raw voltage" {
            }
            frame "Pitot-static tube" {
            }
            frame "Generic Linear" {
            }
            frame "Generic Polynomial" {
            }
            frame "Thermocouple" {
            }
            frame "LDA" {
            }
            frame "Enter Value" {
            }
            frame "ADAM Channel" {
            }
          }
          n200 = Index Array(array=w495) -> (element=w494:string)  [unwired: 1 in]
          n201 = call "Get_Characters_from_string.vi"("Input string"=w497, "Variable name"="An ch 1 Port") -> ("Value"=w493:string)  [unwired: 1 in, 1 out]
          n202 = Bundle By Name(cluster=w490, "Ch"=w491, "DAQ"=w494, "Port"=w493) -> (w496:T14)
          n203 = call "Full Channel ID.vi"("Cluster"=w496) -> ("String"=w492:string)
          n204 = case shown="\"Take a New Calibration Point\", Default" w500 {
            tunnel: w499 -> [w506 w511]
            tunnel: [w506 w510] -> w505
            tunnel: w501 -> [_ w509]
            tunnel: w492 -> [_ w507]
            frame "Refit Curve" {
            }
            frame "Take a New Calibration Point", Default {
              n205 = call "Find_calibration_file.vi"("Inst type"=w509, "Channel ID"=w507, "Use Latest Calib"=FALSE, "filename"=w511) -> ("filename out"=w510:path)
            }
          }
          n206 = Bundle By Name(cluster=w504, "Calib filename"=w505) -> (w503:T10)
        }
      }
      n207 = local write "Reference instrument"(w484) -> ()
    }
    frame #7 {
      # "Get X-wire reference velocity instrument calibration"
      n208 = local read "Ref vel for angle calib"() -> (w525:T7)
      n209 = property on="Ref vel for angle calib" class="Clust (strict)"() -> ("Disabled"=w523:u8)  [unwired: 2 in, 2 out]
      n210 = case shown="0" w523 {
        tunnel: w525 -> [w540 w554]
        tunnel: [w539 w553] -> w524
        tunnel: w522 -> [w526 _]
        frame 0 {
          w536 = FALSE  # Use Latest Calib
          n211 = global read "Meas_global.vi" "Acquisition_Plug_Ins to Run"() -> (w532:string[])
          n212 = Unbundle By Name(w540) -> ("Ref Instrument type"=w538:T3, "Calib filename"=w535:path, "Ch"=w529:i16)
          n213 = global read "Calib_global.vi" "Pre Setup String"() -> (w533:string)
          n214 = case shown="\"Generic Linear\"" w538 {
            tunnel: [Inst_type."Propeller anemometer" ("Inst type") Inst_type."Pressure Transducer" ("Inst type") Inst_type."Pressure Transducer" ("Inst type") Inst_type."Pitot-static tube" ("Inst type") Inst_type."Generic Linear" ("Inst type") Inst_type."Generic Polynomial" ("Inst type") Inst_type."Thermocouple" ("Inst type") Inst_type."Raw voltage" ("Inst type") Inst_type."Raw voltage" ("Inst type") Inst_type."Raw voltage" ("Inst type")] -> w537
            frame "Propellor anemometer" {
            }
            frame "Pressure Transducer" {
            }
            frame "Raw voltage" {
            }
            frame "Pitot-static tube" {
            }
            frame "Generic Linear" {
            }
            frame "Generic Polynomial" {
            }
            frame "Thermocouple" {
            }
            frame "LDA" {
            }
            frame "Enter Value" {
            }
            frame "ADAM Channel" {
            }
          }
          n215 = Index Array(array=w532) -> (element=w531:string)  [unwired: 1 in]
          n216 = call "Get_Characters_from_string.vi"("Input string"=w533, "Variable name"="An ch 1 Port") -> ("Value"=w530:string)  [unwired: 1 in, 1 out]
          n217 = Bundle By Name(cluster=w526, "Ch"=w529, "DAQ"=w531, "Port"=w530) -> (w527:T14)
          n218 = call "Full Channel ID.vi"("Cluster"=w527) -> ("String"=w528:string)
          n219 = call "Find_calibration_file.vi"("Inst type"=w537, "Channel ID"=w528, "Use Latest Calib"=w536, "filename"=w535) -> ("filename out"=w541:path)
          n220 = Bundle By Name(cluster=w540, "Calib filename"=w541) -> (w539:T7)
        }
        frame 1, Default {
          n221 = Bundle By Name(cluster=w554, "Calib filename"=path "") -> (w553:T7)
        }
      }
      n222 = local write "Ref vel for angle calib"(w524) -> ()
    }
    frame #8 {
      w561 = Ref_Inst_type."ADAM Channel" ("Ref Instrument type")
      # "Check if any References channels are ADAM channels"
      n223 = local read "Ref vel for angle calib"() -> (w563:T7)
      n224 = property on="Ref vel for angle calib" class="Clust (strict)"() -> ("Disabled"=w556:u8)  [unwired: 2 in, 2 out]
      n225 = Unbundle By Name(w563) -> ("Ref Instrument type"=w562:T3)
      n226 = Equal To 0?(x=w556) -> (x = 0?=w555:bool)
      n227 = global write "Calib_global.vi" "Ref Instrument type"(w558) -> ()
      n228 = Equal?(x=w561, y=w558) -> (x = y?=w560:bool)
      n229 = local read "2nd ref instrument"() -> (w564:T6)
      n230 = Bundle By Name(cluster=w564, "2nd Ref type"=w562, "2nd inst present"=w555) -> (→"2nd ref instrument":T6)
      n231 = case shown="True" w555 {
        tunnel: w562 -> [_ w570]
        tunnel: w561 -> [_ w569]
        tunnel: w560 -> [w565 w567]
        tunnel: [w565 w566] -> w559
        frame False {
        }
        frame True {
          n232 = Equal?(x=w570, y=w569) -> (x = y?=w568:bool)
          n233 = Or(x=w568, y=w567) -> (x .or. y?=w566:bool)
        }
      }
    }
    frame #9 {
      # "If Reference Inst is an ADAM channel, throw dialogue for user to select channel from"
      n234 = Equal?(x=Calib_mode."Show Setup" ("Mode"), y=w578) -> (x = y?=w577:bool)
      n235 = And(x=w577, y=w576) -> (x .and. y?=w575:bool)
      n236 = global read "Calib_global.vi" "Pre Setup String"() -> (w574:string)
      n237 = case shown="True" w575 {
        tunnel: [w581 w593] -> w579
        tunnel: w574 -> [w583 w592]
        tunnel: "ADAM Channel name" -> [w582 w591]
        tunnel: [w580 w590] -> w572
        frame False {
          n238 = call "Get_Characters_from_string.vi"("Input string"=w583, "Variable name"=w582) -> ("Value"=w580:string)  [unwired: 1 in, 1 out]
          n239 = call "Characters_to_string.vi"("Characters to write"=w580, "Label for characters"=w582) -> ("Output string"=w581:string)  [unwired: 1 in]
        }
        frame True {
          n240 = call "Get_Characters_from_string.vi"("Input string"=w592, "Variable name"=w591) -> ("Status"=w589:enum16{"Char in string", "Char not in string"}, "Value"=w588:string)  [unwired: 1 in]
          n241 = call "Get_ADAM_Ch_names_client.vi"("Channel names set"=Channel_names."Active Only") -> ("Ch names"=w584:string[])
          n242 = case shown="\"Char in string\"" w589 {
            tunnel: w588 -> [w594 _]
            tunnel: [w594 "" ("Value")] -> w587
            frame "Char in string" {
            }
            frame "Char not in string" {
            }
          }
          n243 = call "Select_Single_ADAM_Ch.vi"("Desired Ch name (in)"=w587, "Available Ch names"=w584, "Message"="Please Choose Reference Instrument") -> ("Ch Name"=w590:string)  [unwired: 3 out]
          n244 = call "Characters_to_string.vi"("Characters to write"=w590, "Label for characters"=w591) -> ("Output string"=w593:string)  [unwired: 1 in]
        }
      }
      n245 = global write "Calib_global.vi" "RefADAMChName"(w572) -> ()
    }
    frame #10 {
      # "If Calibated Inst is an ADAM channel, throw dialogue for user to select channel from"
      n246 = local read "InstADAMChName"() -> (w597:string)
      n247 = Equal?(x=Calib_mode."Show Setup" ("Mode"), y=w604) -> (x = y?=w599:bool)
      n248 = Empty String/Path?(string/path=w597) -> (empty?=w600:bool)
      n249 = Compound Arithmetic op=AND(w599, invert w600) -> (w598:bool)
      n250 = global read "Calib_global.vi" "Pre Setup String"() -> (w603:string)
      n251 = case shown="True" w598 {
        tunnel: [w606 w611] -> w596
        tunnel: w603 -> [w608 _]
        tunnel: "1RV:U_ADAM_Ch_Name" -> [w607 w610]
        tunnel: w597 -> [_ w609]
        frame False {
          n252 = call "Get_Characters_from_string.vi"("Input string"=w608, "Variable name"=w607) -> ("Value"=w605:string)  [unwired: 1 in, 1 out]
          n253 = call "Characters_to_string.vi"("Characters to write"=w605, "Label for characters"=w607) -> ("Output string"=w606:string)  [unwired: 1 in]
        }
        frame True {
          n254 = call "Characters_to_string.vi"("Characters to write"=w609, "Label for characters"=w610) -> ("Output string"=w611:string)  [unwired: 1 in]
        }
      }
    }
    frame #11 {
      # "If 2nd reference is ADAM, throw dialogue for user to choose channel"
      n255 = local read "2nd ref instrument"() -> (w618:T6)
      n256 = Equal?(x=Calib_mode."Show Setup" ("Mode"), y=w625) -> (x = y?=w624:bool)
      n257 = global read "Calib_global.vi" "Pre Setup String"() -> (w622:string)
      n258 = Unbundle By Name(w618) -> ("2nd Ref type"=w616:T3, "2nd inst present"=w614:bool)
      n259 = Equal?(x=Ref_Inst_type."ADAM Channel" ("2nd Ref type"), y=w616) -> (x = y?=w615:bool)
      n260 = And(x=w615, y=w614) -> (x .and. y?=w613:bool)
      n261 = And(x=w624, y=w613) -> (x .and. y?=w623:bool)
      n262 = case shown="True" w623 {
        tunnel: [w627 w639] -> w612
        tunnel: w622 -> [w629 w638]
        tunnel: "ADAM Channel name for 2nd Ref Instr" -> [w628 w637]
        tunnel: [w626 w636] -> w620
        frame False {
          n263 = call "Get_Characters_from_string.vi"("Input string"=w629, "Variable name"=w628) -> ("Value"=w626:string)  [unwired: 1 in, 1 out]
          n264 = call "Characters_to_string.vi"("Characters to write"=w626, "Label for characters"=w628) -> ("Output string"=w627:string)  [unwired: 1 in]
        }
        frame True {
          n265 = call "Get_Characters_from_string.vi"("Input string"=w638, "Variable name"=w637) -> ("Status"=w635:enum16{"Char in string", "Char not in string"}, "Value"=w634:string)  [unwired: 1 in]
          n266 = call "Get_ADAM_Ch_names_client.vi"("Channel names set"=Channel_names."Active Only") -> ("Ch names"=w630:string[])
          n267 = case shown="\"Char in string\"" w635 {
            tunnel: w634 -> [w640 _]
            tunnel: [w640 "" ("Value")] -> w633
            frame "Char in string" {
            }
            frame "Char not in string" {
            }
          }
          n268 = call "Select_Single_ADAM_Ch.vi"("Desired Ch name (in)"=w633, "Available Ch names"=w630, "Message"="Please Choose 2nd Ref Channel") -> ("Ch Name"=w636:string)  [unwired: 3 out]
          n269 = call "Characters_to_string.vi"("Characters to write"=w636, "Label for characters"=w637) -> ("Output string"=w639:string)  [unwired: 1 in]
        }
      }
      n270 = global write "Calib_global.vi" "ADAM Channel Name Vel Ref"(w620) -> ()
    }
    frame #12 {
      # "Build up the basic calibration setup string"
      n271 = local read "Reference instrument"() -> (w643:T10)
      n272 = local read "Sampling speeds Output"() -> (w645:T5)
      n273 = local read "2nd ref instrument"() -> (w648:T6)
      n274 = Unbundle By Name(w643) -> ("Ref Instrument type"=w642:T3)
      n275 = Unbundle By Name(w645) -> ("Sampling Rate /ch (Hz)"=w650:sgl, "Samples /ch"=w651:i32)
      n276 = local read "Temp"() -> (w644:dbl)
      n277 = local read "Abs Press"() -> (w646:dbl)
      n278 = global write "Calib_global.vi" "2nd ref instrument"(w648) -> ()
      n279 = global write "Calib_global.vi" "Temp (deg C)"(w644) -> ()
      n280 = call "Calib_General_Setup.vi"("Ref Instrument type"=w642, "Requested No of samples"=w651, "Sampling rate (Hz)"=w650, "2nd ref instrument"=w648, "Temp"=w644, "Abs Press (mbar)"=w646) -> ("Output string"=w649:string, "LDA Data"=w647:bool)  [unwired: 8 out]
      n281 = global write "Calib_global.vi" "Abs Press (mbar)"(w646) -> ()
    }
    frame #13 {
      # "Form strings for X-wire reference channels"
      n282 = local read "Instrument type"() -> (w668:T8)
      n283 = local read "Ref vel for angle calib"() -> (w670:T7)
      n284 = local read "Reference instrument"() -> (w669:T10)
      n285 = global write "Calib_global.vi" "Instrument type"(w668) -> ()
      n286 = case shown="\"Cross wire angle\"" w668 {
        tunnel: [w673 w674 w676] -> w665
        tunnel: w670 -> [w672 w675 _]
        tunnel: [w672 w675 w676] -> w655
        tunnel: w669 -> [w673 w674 w676]
        frame "Propeller anemometer", Default {
        }
        frame "Cross wire angle" {
        }
        frame "Cross wire velocity" {
        }
      }
      n287 = Unbundle By Name(w665) -> ("Calib filename"=w664:path, "Ch"=w663:i16, "Device"=w653:string, "Port"=w662:string, "Ref Instrument type"=w661:T3)  [unwired: 1 out]
      n288 = Unbundle By Name(w655) -> ("Calib filename"=w657:path, "Ch"=w658:i16, "Device"=w652:string, "Port"=w659:string, "Ref Instrument type"=w660:T3)  [unwired: 1 out]
      n289 = call "Reference_Inst_Info_2_string.vi"("Ref Instrument type"=w661, "Calib filename"=w664, "Port"=w662, "Device"=w653, "Ch No"=w663, "Reference Name"="Reference instrument") -> ("Setup String"=w666:string)
      n290 = call "Reference_Inst_Info_2_string.vi"("Ref Instrument type"=w660, "Calib filename"=w657, "Port"=w659, "Device"=w652, "Ch No"=w658, "Reference Name"="Ref vel for angle calib") -> ("Setup String"=w654:string)
      n291 = Concatenate Strings(w666, w654) -> (w671:string)
    }
    frame #14 {
      # "Throw Pulsed Wire setup panel, if running PWA, and form string"
      n292 = local read "Instrument type"() -> (w677:T8)
      n293 = case shown="\"Pulsed Wire\"" w677 {
        tunnel: ["" w686] -> w678
        tunnel: w679 -> [_ w685]
        frame "Propeller anemometer", Default {
        }
        frame "Pulsed Wire" {
          w681 = FALSE  # Check Calib file?
          n294 = case shown="\"Show Setup\"" w685 {
            tunnel: [w688 w690] -> w684
            tunnel: [w687 w689] -> w683
            frame "Refit Curve", Default {
              w688 = FALSE  # Show Panel?
              w687 = T13 TRUE  # OK
            }
            frame "Show Setup" {
              w690 = TRUE  # Show Panel?
              w689 = T13 FALSE  # OK
            }
          }
          n295 = global read "Calib_global.vi" "Pre Setup String"() -> (w682:string)
          n296 = call "PWA_Setup_Panel.vi"("Show Panel?"=w684, "Check Calib file?"=w681, "OK"=w683, "Incoming Setup String"=w682) -> ("Outgoing Setup String"=w686:string)  [unwired: 3 out]
        }
      }
    }
    frame #15 {
      # "Form channels and spans string"
      n297 = local read "instrument to calibrate"() -> (w693:T11)
      n298 = for {
        tunnel: w693 -> [w720] mode=indexing
        shift-right: [w714] -> w696
        shift-left: "" -> [w715]
        i -> [w719]
        n299 = Unbundle By Name(w720) -> ("Acquisition Plug in"=w702:string, "Port"=w706:string, "Ch No"=w716:i16)
        n300 = Increment(x=w719) -> (x+1=w713:i32)
        n301 = Format Into String(format string="Inst_to_calibrate_element_%d ", w713) -> (resulting string=w707:string)  [unwired: 2 in, 1 out]
        n302 = Concatenate Strings(w707, "Ch No") -> (w718:string)
        n303 = Concatenate Strings(w707, "Device") -> (w708:string)
        n304 = Concatenate Strings(w707, "Port") -> (w711:string)
        n305 = call "Characters_to_string.vi"("Characters to write"=w702, "Label for characters"=w708) -> ("Output string"=w705:string)  [unwired: 1 in]
        n306 = call "Characters_to_string.vi"("Characters to write"=w706, "Label for characters"=w711) -> ("Output string"=w704:string)  [unwired: 1 in]
        n307 = call "Value_to_string.vi"("Value"=w716, "Label for value"=w718) -> ("Output string"=w703:string)  [unwired: 1 in]
        n308 = Concatenate Strings(w715, w705, w704, w703) -> (w714:string)
      }
      n309 = Array Size(array=w693) -> (size(s)=w692:i32)
      n310 = Equal To 0?(x=w692) -> (x = 0?=w691:bool)
      n311 = case shown="False" w691 {
        tunnel: [w698 i16 -10 ("Ch No")] -> w694
        tunnel: w693 -> [w697 _]
        frame False {
          w700 = 0  # index
          n312 = Index Array(array=w697, index=w700) -> (element=w699:T23)
          n313 = Unbundle By Name(w699) -> ("Ch No"=w698:i16)
        }
        frame True {
        }
      }
      n314 = global write "Calib_global.vi" "Calib Ch No"(w694) -> ()
    }
    frame #16 {
      # "Assemble the calibration setup string"
      n315 = global write "Calib_global.vi" "zeroable?"("zeroable?") -> ()
      n316 = local read "Fixed n out"() -> (w742:bool)
      n317 = case shown="\"Zeroable\"" "zeroable?" {
        tunnel: ["TRUE" "FALSE"] -> w724
        frame "Zeroable" {
        }
        frame "Do Not Zero" {
        }
      }
      n318 = Select(t="TRUE", s=w742, f="FALSE") -> (s? t:f=w743:string)
      n319 = local read "Instrument type"() -> (w737:T8)
      n320 = property on="Instrument type" class="Enum (strict)"() -> ("Strings []"=w738:string[])  [unwired: 2 in, 2 out]
      n321 = property on="angle calib" class="Enum (strict)"() -> ("Strings []"=w733:string[])  [unwired: 2 in, 2 out]
      n322 = local read "angle calib"() -> (w732:T9)
      n323 = Index Array(array=w738, index=w737) -> (element=w736:string)
      n324 = Index Array(array=w733, index=w732) -> (element=w731:string)
      n325 = call "Characters_to_string.vi"("Characters to write"=w724, "Label for characters"="Zeroable") -> ("Output string"=w721:string)  [unwired: 1 in]
      n326 = call "Characters_to_string.vi"("Characters to write"=w731, "Label for characters"="Angle calib") -> ("Output string"=w727:string)  [unwired: 1 in]
      n327 = call "Characters_to_string.vi"("Characters to write"=w736, "Label for characters"="Instrument_type_to Calibrate") -> ("Output string"=w722:string)  [unwired: 1 in]
      n328 = call "Characters_to_string.vi"("Characters to write"=w743, "Label for characters"="Fixed Coefficient n") -> ("Output string"=w739:string)  [unwired: 1 in]
      n329 = global read "Calib_global.vi" "New Setup String"() -> (w741:string)
      n330 = Concatenate Strings(w741, w739, w721, w722, w727, w748, w726, w728, w747, w729, w740, w730) -> (w749:string)
      n331 = global write "Calib_global.vi" "New Setup String"(w749) -> ()
    }
    frame #17 {
      # "Throw the BSA setup"
      n332 = Equal?(x=Calib_mode."Show Setup" ("Mode"), y=w757) -> (x = y?=w756:bool)
      n333 = And(x=w755, y=w756) -> (x .and. y?=w754:bool)
      n334 = case shown="True" w754 {
        tunnel: [FALSE ("Synchronise with LDA") FALSE ("Synchronise with LDA")] -> w752
        frame False {
        }
        frame True {
          n335 = call "Edit LDA Setup.vi"("LDA info in Setup File?"=TRUE) -> ()  [unwired: 11 in]
        }
      }
      n336 = global write "Meas_global.vi" "Use  Analogue channel to software sync with LDA"(w752) -> ()
    }
    frame #18 {
      # "Assembles \"Calib_Setup\" file from portions of the calibration setup string to provide setup for measurement program"
      n337 = global read "Meas_global.vi" "LDA data"() -> (w762:enum16{"No LDA data", "Take LDA data"})
      n338 = local read "Instrument type"() -> (w769:T8)
      n339 = local read "Ch & spans"() -> (w772:T12[])
      n340 = local read "Calib filename"() -> (w780:path)
      n341 = case shown="\"Pulsed Wire\"" w769 {
        tunnel: ["" w789] -> w768
        frame "Propeller anemometer", Default {
        }
        frame "Pulsed Wire" {
          n342 = property on="PWA Data" class="Enum (strict)"() -> ("Strings []"=w792:string[])  [unwired: 2 in, 2 out]
          n343 = Index Array(array=w792, index=PWA_Data."One Ch PWA" ("PWA Data")) -> (element=w790:string)
          n344 = call "Characters_to_string.vi"("Characters to write"=w790, "Label for characters"="Pulsed_Wire_Data" ("Variable name")) -> ("Output string"=w789:string)  [unwired: 1 in]
        }
      }
      n345 = case shown="\"Take LDA data\"" w762 {
        tunnel: ["" w782] -> w761
        frame "No LDA data" {
        }
        frame "Take LDA data" {
          n346 = global read "Constants_global.vi" "All_Users"() -> (w786:path)
          n347 = Build Path(base path=w786, name or relative path="LDA_Setup") -> (appended path=w785:path)
          n348 = Build Path(base path=w785, name or relative path="LDA_Setup_File.xls") -> (appended path=w783:path)
          n349 = Read from Text File(file (use dialog)=w783) -> (text=w782:string)  [unwired: 3 in, 3 out]
        }
      }
      n350 = call "Calib_Ch_setup.vi"("Ch & spans"=w772, "Calib filename"=w780) -> ("Output string"=w773:string)  [unwired: 4 in]
      n351 = global write "Calib_global.vi" "Ref Calib file"(w780) -> ()
      n352 = global write "Calib_global.vi" "Ch & spans"(w772) -> ()
      n353 = call "Date_and_Time_to_string.vi"() -> ("Date and time (spreadsheet)"=w771:string)  [unwired: 4 in, 1 out]
      n354 = Concatenate Strings(w771, w768, w761, w774, w763, w773, w767) -> (w775:string)
      n355 = call "Add_label_to_string.vi"("String to write"=w775, "File Label"="Raw data header") -> ("Output string"=w776:string)
      n356 = call "Setup_Filepath.vi"("Setup File Type"=Setup_Filetype."Measurement Setups", "Filename in"="Calib_Setup.xls") -> ("Filename Out"=w764:path)  [unwired: 1 out]
      n357 = call "Write_Characters_To_File.vi"("file path (dialog if empty)"=w764, "advisory dialog? (display:T)"=FALSE, "character string"=w776, "append to file? (new file:F)"=FALSE, "Lock File"=TRUE) -> ()  [unwired: 4 out]
    }
    frame #19 {
      # "Closes itself when done"
      n358 = case shown="\"Show Setup\"" w794 {
        frame "Show Setup" {
          n359 = Current VI's Path() -> (path=w796:path)
          n360 = call "Open_Close_Front_Panel.ph.vi"("openWindow (T)"=FALSE ("Front Panel Window:Open"), "VI path"=w796) -> ()  [unwired: 1 in, 1 out]
        }
        frame "Take a New Calibration Point", Default {
        }
      }
    }
  }
